vi "Motion_3D_RecordWaveform_win7.vi"() -> ()   [LabVIEW 2017]
panel:
  in  "resource name 2":refnum<k15> caption="resource name"
  out "Path To File Info":path
  out "Path To File":path
  in  "File Name":path
  in  "2^9 Averages":i32=2 min=1 max=9 step=1
  in  "Decimation Factor":i32=1 min=1 max=1000
  out "Sampling Frequency (MHz)":dbl
  out "Number of Averages":i32
  in  "Averaging On or Off":bool
  in  "Stop Time (us)":dbl
  in  "Start Time (us)":dbl
  out "XY Graph":cluster{"Y":dbl[], "Y":dbl[]}[](graph)
  in  "Third Motor\nNumber":i32=1 min=1 max=3 step=1
  in  "Step Size \nThird  (um)":dbl
  in  "Raster Scan Length \nThird  (mm)":dbl
  in  "Primary Motor\nNumber":i32=1 min=1 max=3 step=1
  in  "Secondary Motor\nNumber":i32=1 min=1 max=3 step=1
  in  "Motor Speed (mm/sec)":dbl=10.0 caption="Range:0.1-30 by 0.1" min=0.1 max=30.0 step=0.1
  in  "Step Size \nPrimary (um)":dbl
  in  "Raster Scan Length \nPrimary (mm)":dbl
  in  "Step Size \nSecondary  (um)":dbl
  in  "Raster Scan Length \nSecondary  (mm)":dbl
  in  "Operation":string(combo)
  in  "Single Axis Movement":dbl caption="(mm)"
  in  "Motor Number":i32=1 min=1 max=3 step=1
  # "Primary Scan Length MUST be >0\nSecondary Scan Length Must be > or = 0"
  # "+3"
  # "+2"
  # "+1"
  # "MOTION CONTROL"
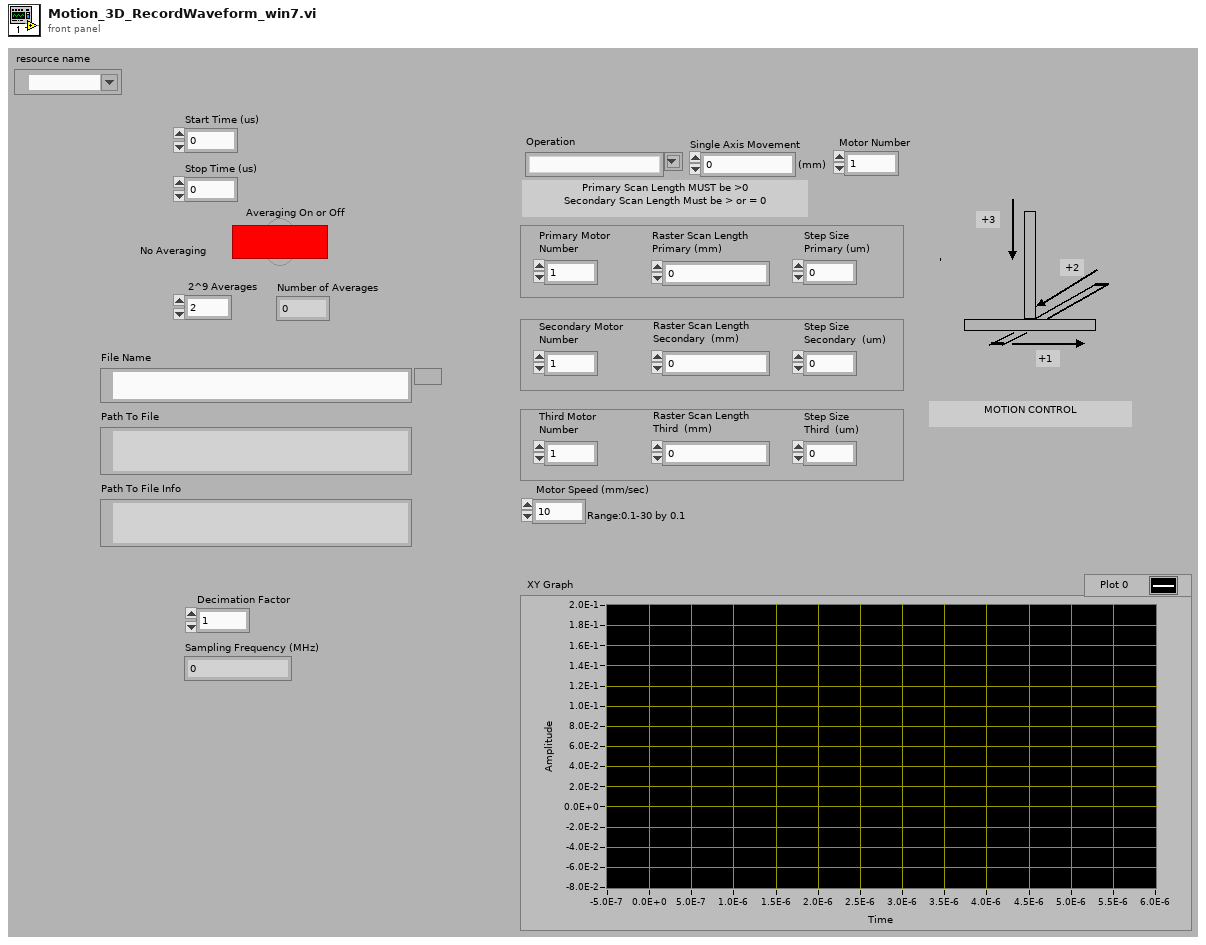
[diagram p1: front panel]
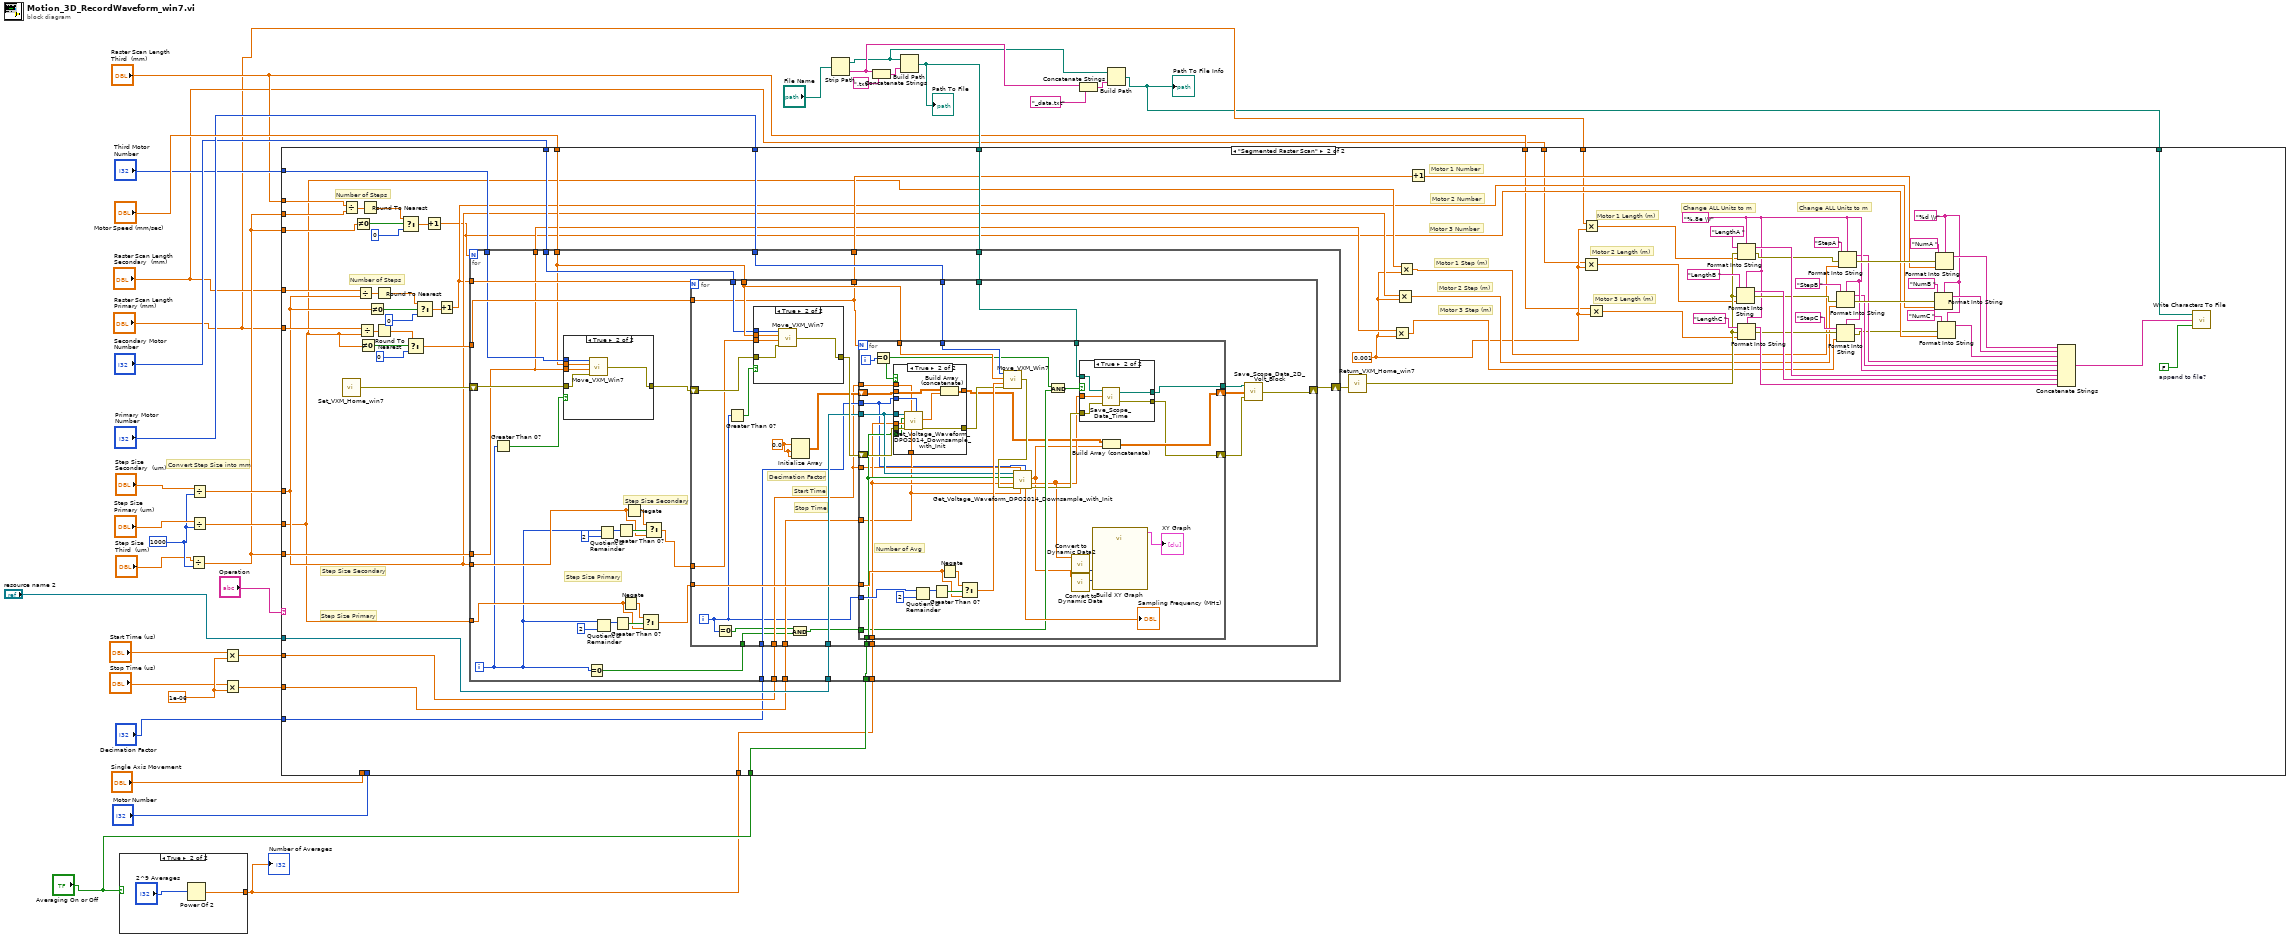
[diagram p0: block diagram]
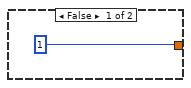
[diagram p2: hidden frame]
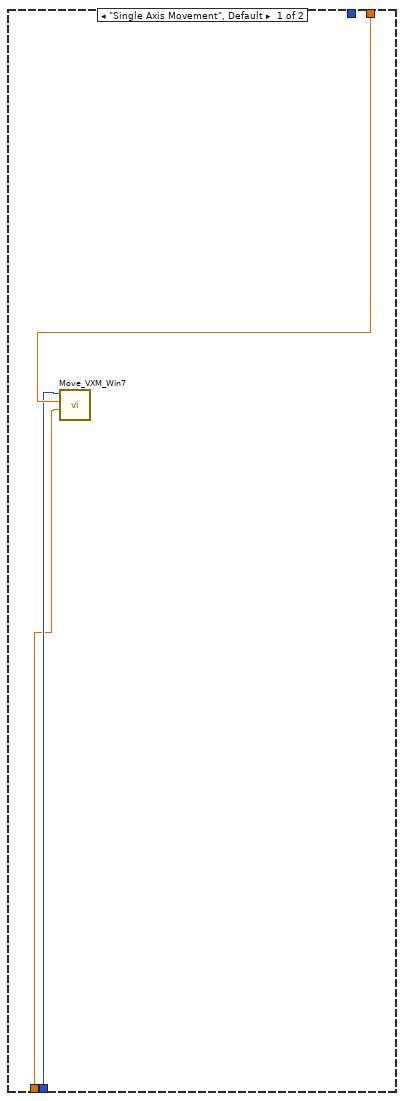
[diagram p3: hidden frame]
diagram:
  w19 = 1e-06
  w25 = 1000
  # "Convert Step Size into mm"
  n1 = case shown="True" "Averaging On or Off" {
    tunnel: [1 w38] -> w20
    frame False {
    }
    frame True {
      n2 = Power Of 2(x="2^9 Averages") -> (2^x=w38:dbl)
    }
  }
  "Number of Averages" <- w20
  n3 = Divide(x="Step Size \nThird  (um)", y=w25) -> (x/y=w22:dbl)
  n4 = Divide(x="Step Size \nSecondary  (um)", y=w25) -> (x/y=w28:dbl)
  n5 = Divide(x="Step Size \nPrimary (um)", y=w25) -> (x/y=w29:dbl)
  n6 = Multiply(x="Start Time (us)", y=w19) -> (x*y=w16:dbl)
  n7 = Multiply(x="Stop Time (us)", y=w19) -> (x*y=w15:dbl)
  n8 = Strip Path(path="File Name") -> (stripped path=w7:path, name=w8:string)
  n9 = Concatenate Strings(w8, ".txt") -> (w12:string)
  n10 = Build Path(base path=w7, name or relative path=w12) -> (appended path=w6:path)
  "Path To File" <- w6
  n11 = Concatenate Strings(w8, "_data.txt") -> (w9:string)
  n12 = Build Path(base path=w7, name or relative path=w9) -> (appended path=w2:path)
  "Path To File Info" <- w2
  n13 = case shown="\"Segmented Raster Scan\"" "Operation" {
    tunnel: "Raster Scan Length \nSecondary  (mm)" -> [_ w120]
    tunnel: "Raster Scan Length \nPrimary (mm)" -> [_ w119]
    tunnel: w28 -> [_ w86]
    tunnel: w29 -> [_ w85]
    tunnel: "Motor Speed (mm/sec)" -> [w41 w122]
    tunnel: "Primary Motor\nNumber" -> [_ w121]
    tunnel: "Motor Number" -> [w40 _]
    tunnel: "Single Axis Movement" -> [w39 _]
    tunnel: "Secondary Motor\nNumber" -> [_ w117]
    tunnel: "Raster Scan Length \nThird  (mm)" -> [_ w101]
    tunnel: w22 -> [_ w100]
    tunnel: "Third Motor\nNumber" -> [_ w99]
    tunnel: w22 -> [_ w98]
    tunnel: w22 -> [_ w97]
    tunnel: "Averaging On or Off" -> [_ w95]
    tunnel: w20 -> [_ w94]
    tunnel: "resource name 2" -> [_ w93]
    tunnel: w16 -> [_ w92]
    tunnel: w15 -> [_ w91]
    tunnel: "Decimation Factor" -> [_ w90]
    tunnel: w6 -> [_ w89]
    tunnel: "Raster Scan Length \nThird  (mm)" -> [_ w48]
    tunnel: "Raster Scan Length \nSecondary  (mm)" -> [_ w47]
    tunnel: "Raster Scan Length \nPrimary (mm)" -> [_ w46]
    tunnel: w2 -> [_ w43]
    frame "Single Axis Movement", Default {
      n14 = call "Move_VXM_Win7.vi"("Single Axis Movement (mm)"=w39, "Motor Speed (mm/sec)"=w41, "Motor Number"=w40) -> ()  [unwired: 1 in, 1 out]
    }
    frame "Segmented Raster Scan" {
      w45 = FALSE  # append to file?
      w42 = "%d \\r" ("format string")
      w67 = "%.8e \\r"
      w49 = 0.001
      # "Motor 3 Length (m)"
      # "Motor 2 Length (m)"
      # "Motor 1 Length (m)"
      # "Change ALL Units to m"
      # "Change ALL Units to m"
      # "Motor 3 Step (m)"
      # "Motor 2 Step (m)"
      # "Motor 1 Step (m)"
      # "Motor 3 Number"
      # "Motor 2 Number"
      # "Motor 1 Number"
      # "Step Size Primary"
      # "Step Size Secondary"
      # "Number of Steps"
      # "Number of Steps"
      n15 = call "Set_VXM_Home_win7.vi"() -> ("error out"=w96:errorcluster)  [unwired: 1 in]
      n16 = Divide(x=w101, y=w100) -> (x/y=w106:dbl)
      n17 = Not Equal To 0?(x=w97) -> (x != 0?=w105:bool)
      n18 = Divide(x=w120, y=w86) -> (x/y=w115:dbl)
      n19 = Divide(x=w119, y=w85) -> (x/y=w116:dbl)
      n20 = Not Equal To 0?(x=w85) -> (x != 0?=w114:bool)
      n21 = Round To Nearest(number=w106) -> (nearest integer value=w103:dbl)
      n22 = Not Equal To 0?(x=w86) -> (x != 0?=w111:bool)
      n23 = Round To Nearest(number=w115) -> (nearest integer value=w109:dbl)
      n24 = Round To Nearest(number=w116) -> (nearest integer value=w113:dbl)
      n25 = Select(t=w103, s=w105, f=0) -> (s? t:f=w102:dbl)
      n26 = Select(t=w113, s=w114, f=0) -> (s? t:f=w107:dbl)
      n27 = Select(t=w109, s=w111, f=0) -> (s? t:f=w108:dbl)
      n28 = Increment(x=w102) -> (x+1=w54:dbl)
      n29 = Increment(x=w108) -> (x+1=w55:dbl)
      n30 = for {
        N: w54 -> [_]
        tunnel: w122 -> [w148]
        tunnel: w121 -> [w155]
        tunnel: w85 -> [w136]
        tunnel: w117 -> [w153]
        tunnel: w107 -> [w152]
        tunnel: w55 -> [w151]
        tunnel: w86 -> [w134]
        shift-right: [w154] -> w118
        shift-left: w96 -> [w147]
        tunnel: w99 -> [w149]
        tunnel: w98 -> [w123]
        tunnel: w95 -> [w133]
        tunnel: w94 -> [w132]
        tunnel: w93 -> [w131]
        tunnel: w92 -> [w130]
        tunnel: w91 -> [w129]
        tunnel: w90 -> [w128]
        tunnel: w89 -> [w125]
        tunnel: [w124] -> w88
        tunnel: [w123] -> w87
        i -> [w127]
        # "Step Size Primary"
        # "Step Size Secondary"
        n31 = Greater Than 0?(x=w127) -> (x > 0?=w150:bool)
        n32 = case shown="True" w150 {
          tunnel: [w156 w158] -> w146
          tunnel: w147 -> [w156 w157]
          tunnel: w123 -> [_ w161]
          tunnel: w148 -> [_ w159]
          tunnel: w149 -> [_ w160]
          frame False {
          }
          frame True {
            n33 = call "Move_VXM_Win7.vi"("error in (no error)"=w157, "Single Axis Movement (mm)"=w161, "Motor Speed (mm/sec)"=w159, "Motor Number"=w160) -> ("error out"=w158:errorcluster)
          }
        }
        n34 = Equal To 0?(x=w127) -> (x = 0?=w126:bool)
        n35 = Quotient & Remainder(x=w127, y=2) -> (x-y*floor(x/y)=w144:i32)  [unwired: 1 out]
        n36 = Quotient & Remainder(x=w127, y=2) -> (x-y*floor(x/y)=w140:i32)  [unwired: 1 out]
        n37 = Greater Than 0?(x=w144) -> (x > 0?=w143:bool)
        n38 = Greater Than 0?(x=w140) -> (x > 0?=w139:bool)
        n39 = Negate(x=w136) -> (-x=w142:dbl)
        n40 = Negate(x=w134) -> (-x=w138:dbl)
        n41 = Select(t=w142, s=w143, f=w136) -> (s? t:f=w135:dbl)
        n42 = Select(t=w138, s=w139, f=w134) -> (s? t:f=w137:dbl)
        n43 = for {
          N: w151 -> [_]
          tunnel: w148 -> [w182]
          shift-right: [w165] -> w154
          shift-left: w146 -> [w184]
          tunnel: w137 -> [w183]
          tunnel: w152 -> [w162]
          tunnel: w155 -> [w187]
          tunnel: w135 -> [w186]
          tunnel: w153 -> [w181]
          tunnel: w133 -> [w178]
          tunnel: w132 -> [w177]
          tunnel: w131 -> [w175]
          tunnel: w130 -> [w172]
          tunnel: w129 -> [w174]
          tunnel: w128 -> [w173]
          tunnel: w126 -> [w169]
          tunnel: w125 -> [w164]
          tunnel: [w162] -> w124
          i -> [w171]
          w179 = 0.0
          # "Decimation Factor"
          # "Stop Time"
          # "Start Time"
          n44 = Equal To 0?(x=w171) -> (x = 0?=w170:bool)
          n45 = Greater Than 0?(x=w171) -> (x > 0?=w185:bool)
          n46 = case shown="True" w185 {
            tunnel: [w188 w190] -> w180
            tunnel: w184 -> [w188 w189]
            tunnel: w183 -> [_ w193]
            tunnel: w182 -> [_ w192]
            tunnel: w181 -> [_ w191]
            frame False {
            }
            frame True {
              n47 = call "Move_VXM_Win7.vi"("error in (no error)"=w189, "Single Axis Movement (mm)"=w193, "Motor Speed (mm/sec)"=w192, "Motor Number"=w191) -> ("error out"=w190:errorcluster)
            }
          }
          n48 = And(x=w170, y=w169) -> (x .and. y?=w168:bool)
          n49 = Initialize Array(w179, w179, w179) -> (w176:dbl[][])
          n50 = for {
            N: w162 -> [_]
            tunnel: w182 -> [w224]
            tunnel: w187 -> [w223]
            tunnel: w186 -> [w225]
            tunnel: w171 -> [w221]
            shift-right: [w196] -> w166
            shift-left: w180 -> [w219]
            tunnel: w178 -> [w213]
            tunnel: w177 -> [w212]
            shift-right: [w202] -> w167
            shift-left: w176 -> [w217]
            tunnel: w175 -> [w214]
            tunnel: w172 -> [w216]
            tunnel: w174 -> [w210]
            tunnel: w173 -> [w209]
            tunnel: w172 -> [w211]
            tunnel: w168 -> [w205]
            tunnel: w164 -> [w195]
            tunnel: [w194] -> w163
            i -> [w218]
            # "Number of Avg"
            n51 = Equal To 0?(x=w218) -> (x = 0?=w206:bool)
            n52 = case shown="True" w206 {
              tunnel: w214 -> [_ w244]
              tunnel: w212 -> [_ w245]
              tunnel: w219 -> [w238 w246]
              tunnel: [w238 w247] -> w220
              tunnel: [w237 w248] -> w203
              tunnel: w217 -> [w237 w249]
              tunnel: w209 -> [_ w242]
              tunnel: w213 -> [_ w241]
              tunnel: w216 -> [_ w240]
              tunnel: w210 -> [_ w239]
              frame False {
              }
              frame True {
                n53 = call "Get_Voltage_Waveform_DPO2014_Downsample_with_Init.vi"("Decimation Factor"=w242, "Stop Time"=w239, "Start Time"=w240, "error in (no error)"=w246, "Number of Averages"=w245, "Averaging On or Off"=w241, "resource name"=w244) -> ("error out"=w247:errorcluster, "Voltage Down Sample"=w243:dbl[])  [unwired: 3 out]
                n54 = Build Array (concatenate)(w249, w243) -> (w248:dbl[][])
              }
            }
            n55 = Quotient & Remainder(x=w221, y=2) -> (x-y*floor(x/y)=w228:i32)  [unwired: 1 out]
            n56 = Greater Than 0?(x=w228) -> (x > 0?=w227:bool)
            n57 = Negate(x=w225) -> (-x=w226:dbl)
            n58 = Select(t=w226, s=w227, f=w225) -> (s? t:f=w222:dbl)
            n59 = call "Move_VXM_Win7.vi"("error in (no error)"=w220, "Single Axis Movement (mm)"=w222, "Motor Speed (mm/sec)"=w224, "Motor Number"=w223) -> ("error out"=w215:errorcluster)
            n60 = call "Get_Voltage_Waveform_DPO2014_Downsample_with_Init.vi"("Decimation Factor"=w209, "Stop Time"=w210, "Start Time"=w211, "error in (no error)"=w215, "Number of Averages"=w212, "Averaging On or Off"=w213, "resource name"=w214) -> ("error out"=w204:errorcluster, "Time Down Sample"=w198:dbl[], "Voltage Down Sample"=w197:dbl[], "Sampling Frequency (MHz)"=→"Sampling Frequency (MHz)":dbl)  [unwired: 1 out]
            n61 = And(x=w206, y=w205) -> (x .and. y?=w207:bool)
            n62 = call "Convert to Dynamic Data2"("Array"=w198) -> ("Dynamic Data Type"=w201:dynamicdata)  [unwired: 3 in]
            n63 = call "Convert to Dynamic Data"("Array"=w197) -> ("Dynamic Data Type"=w200:dynamicdata)  [unwired: 3 in]
            n64 = case shown="True" w207 {
              tunnel: w204 -> [w230 w235]
              tunnel: w198 -> [_ w236]
              tunnel: w195 -> [w231 w234]
              tunnel: [w230 w233] -> w196
              tunnel: [w231 w232] -> w194
              frame False {
              }
              frame True {
                n65 = call "Save_Scope_Data_Time.vi"("error in (no error)"=w235, "Time"=w236, "Path"=w234) -> ("error out"=w233:errorcluster, "Path 2"=w232:path)
              }
            }
            n66 = call "Build XY Graph"("Y Input"=w200, "X Input"=w201) -> ("XY Graph"=→"XY Graph":cluster{"Y":dbl[], "Y":dbl[]}[])  [unwired: 8 in, 1 out]
            n67 = Build Array (concatenate)(w203, w197) -> (w202:dbl[][])
          }
          n68 = call "Save_Scope_Data_2D_Volt_Block.vi"("error in (no error)"=w166, "Voltage"=w167, "Path"=w163) -> ("error out"=w165:errorcluster)
        }
      }
      n69 = call "Return_VXM_Home_win7.vi"("error in (no error)"=w118) -> ("error out"=w71:errorcluster)
      n70 = Multiply(x=w87, y=w49) -> (x*y=w63:dbl)
      n71 = Multiply(x=w86, y=w49) -> (x*y=w62:dbl)
      n72 = Multiply(x=w85, y=w49) -> (x*y=w61:dbl)
      n73 = Increment(x=w88) -> (x+1=w56:dbl)
      n74 = Multiply(x=w47, y=w49) -> (x*y=w51:dbl)
      n75 = Multiply(x=w46, y=w49) -> (x*y=w52:dbl)
      n76 = Multiply(x=w48, y=w49) -> (x*y=w50:dbl)
      n77 = Format Into String "Format Into String"(format string=w67, initial string="LengthB ", error in=w71, w51) -> (resulting string=w78:string, error out=w75:errorcluster)
      n78 = Format Into String "Format Into String"(format string=w67, initial string="LengthA ", error in=w71, w52) -> (resulting string=w77:string, error out=w76:errorcluster)
      n79 = Format Into String "Format Into String"(format string=w67, initial string="LengthC ", error in=w71, w50) -> (resulting string=w70:string, error out=w69:errorcluster)
      n80 = Format Into String "Format Into String"(format string=w67, initial string="StepB ", error in=w75, w62) -> (resulting string=w65:string, error out=w73:errorcluster)
      n81 = Format Into String "Format Into String"(format string=w67, initial string="StepC ", error in=w69, w63) -> (resulting string=w66:string, error out=w53:errorcluster)
      n82 = Format Into String "Format Into String"(format string=w67, initial string="StepA ", error in=w76, w61) -> (resulting string=w64:string, error out=w74:errorcluster)
      n83 = Format Into String "Format Into String"(format string=w42, initial string="NumB ", error in=w73, w55) -> (resulting string=w58:string)  [unwired: 1 out]
      n84 = Format Into String "Format Into String"(format string=w42, initial string="NumA ", error in=w74, w56) -> (resulting string=w57:string)  [unwired: 1 out]
      n85 = Format Into String "Format Into String"(format string=w42, initial string="NumC ", error in=w53, w54) -> (resulting string=w59:string)  [unwired: 1 out]
      n86 = Concatenate Strings(w57, w58, w59, w64, w65, w66, w77, w78, w70) -> (w44:string)
      n87 = call <vilib>:"Write Characters To File.vi"("append to file? (new file:F)"=w45, "character string"=w44, "file path (dialog if empty)"=w43) -> ()  [unwired: 2 in, 1 out]
    }
  }
